vi "Write DMM classes.vi"(10 "DMM classes":refnum<class "Digital Multimeter.lvclass">[](array[class]), 11 "Measurements in":refnum<class "Measurement.lvclass">) -> (3 "Measurements out":refnum<class "Measurement.lvclass">)   [LabVIEW 2020, in "Measurement.lvclass"]
uses:
  Measurement.lvclass
  Instruments/Digital Multimeter/Digital Multimeter.lvclass
  Measurement.lvclass/Measurement.ctl
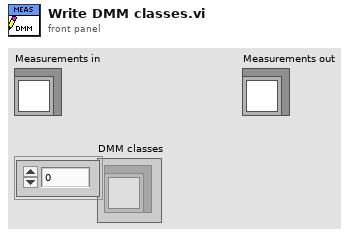
[diagram p1: front panel]
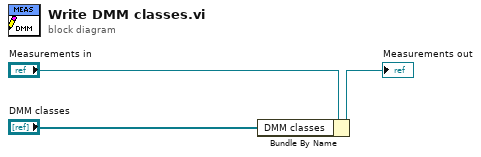
[diagram p0: block diagram]
diagram:
  n1 = Bundle By Name(cluster="Measurements in", "DMM classes"="DMM classes") -> (→"Measurements out":refnum<class "Measurement.lvclass">)
